vi "Write Use Tiered Panels_.vi"(8 "error in (no error)":errorcluster, 10 "Use Tiered Panels?":bool, 11 "Panel Form Controller Configuration in":refnum<class "Panel Form Controller Configuration.lvclass">) -> (0 "error out":errorcluster, 3 "Panel Form Controller Configuration out":refnum<class "Panel Form Controller Configuration.lvclass">)   [LabVIEW 2020, in "Panel Form Controller.lvlib" / "Panel Form Controller Configuration.lvclass"]
uses:
  Panel Form Controller Configuration.lvclass
  Panel Form Controller Configuration.lvclass/Panel Form Controller Configuration.ctl
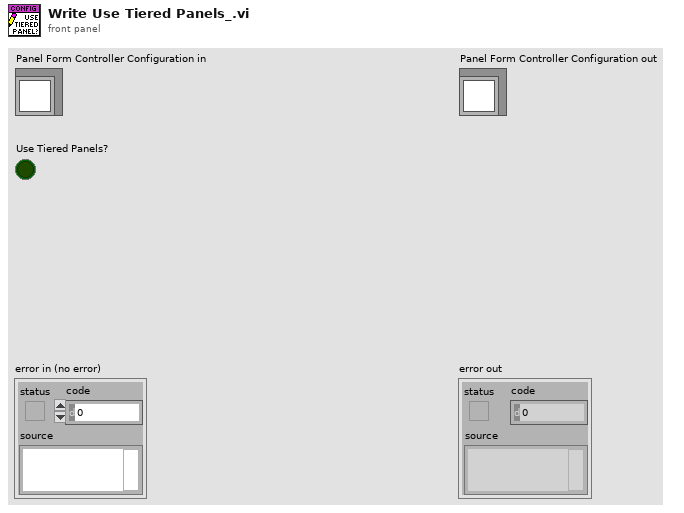
[diagram p1: front panel]
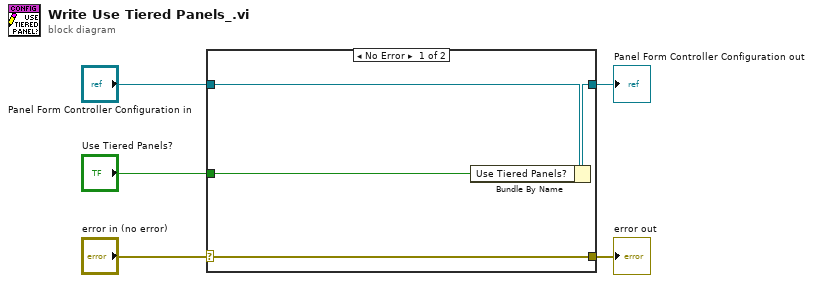
[diagram p0: block diagram]
diagram:
  n1 = case shown="No Error" "error in (no error)" {
    selector: "error in (no error)" -> [w9 w10]
    tunnel: [w9 w10] -> w4
    tunnel: [w7 w11] -> w2
    tunnel: "Panel Form Controller Configuration in" -> [w8 w11]
    tunnel: "Use Tiered Panels?" -> [w6 _]
    frame No Error {
      n2 = Bundle By Name(cluster=w8, "Use Tiered Panels?"=w6) -> (w7:refnum<class "Panel Form Controller Configuration.lvclass">)
    }
    frame Error {
    }
  }
  "error out" <- w4
  "Panel Form Controller Configuration out" <- w2
